vi "DAQStartRec.vi"(4 "entrée d'erreur (pas d'erreur)":errorcluster, 6 "ConfigurationTotale":T1, 7 "path out":path) -> (0 "sortie d'erreur":errorcluster, 3 "Refnum en sortie":refnum<k21>)   [LabVIEW 2015]
uses:
  DefDeType/ConfigTotale.ctl
  DefDeType/VoltageChannels.ctl
  DefDeType/WBridgeChannels.ctl
  DefDeType/Configuration.ctl
  <vilib>/DAQmx/configure/task.llb/DAQmx Configure Logging (TDMS).vi
  <vilib>/DAQmx/configure/trigger.llb/DAQmx Start Trigger (Digital Edge).vi
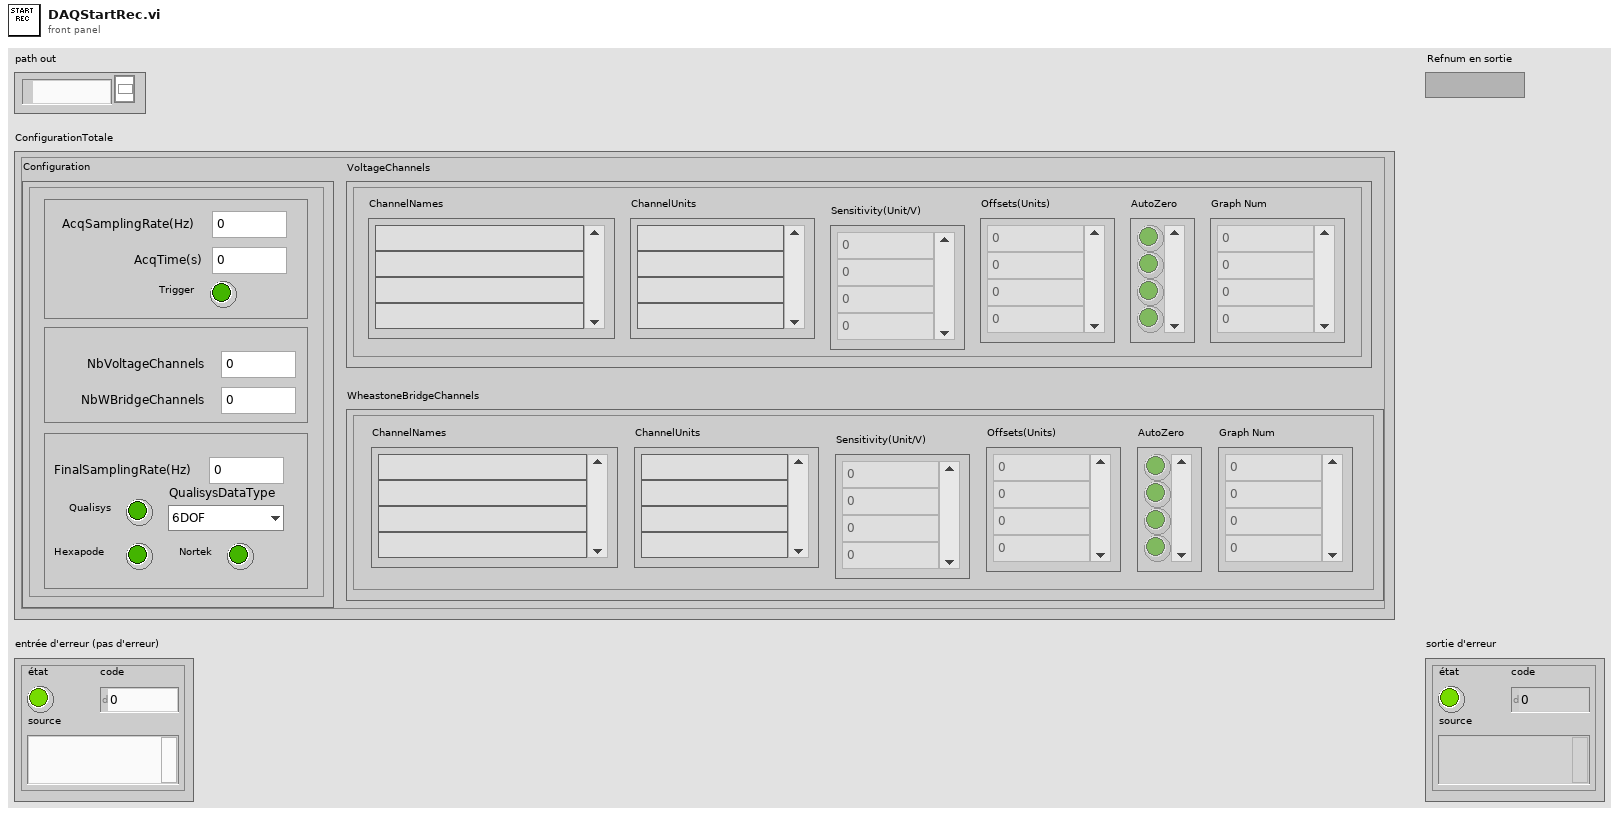
[diagram p1: front panel]
types:
  T1 = typedef "ConfigTotale.ctl" = cluster{"VoltageChannels":T2, "WheastoneBridgeChannels":T3, "Configuration":T4}
  T2 = typedef "VoltageChannels.ctl" = cluster{"ChannelNames":string[], "Sensitivity(Unit/V)":dbl[], "AutoZero":bool[], "ChannelUnits":string[], "Offsets(Units)":dbl[], "Graph Num":u8[]}
  T3 = typedef "WBridgeChannels.ctl" = cluster{"ChannelNames":string[], "Sensitivity(Unit/V)":dbl[], "AutoZero":bool[], "ChannelUnits":string[], "Offsets(Units)":dbl[], "Graph Num":u8[]}
  T4 = typedef "Configuration.ctl" = cluster{"AcqSamplingRate(Hz)":u32, "AcqTime(s)":u32, "Trigger":bool, "NbVoltageChannels":u32, "NbWBridgeChannels":u32, "Qualisys":bool, "Hexapode":bool, "FinalSamplingRate(Hz)":u32, "QualisysDataType":enum16{"6DOF", "3DTracking"}, "Nortek":bool}
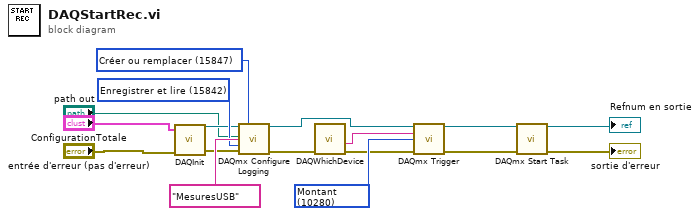
[diagram p0: block diagram]
diagram:
  w16 = 10280 items=["Montant"=10280, "Descendant"=10171] ("edge")
  w8 = 15847 items=["Ouvrir"=10437, "Ouvrir ou créer"=15846, "Créer ou remplacer"=15847, "Créer"=15848] ("operation")
  w7 = 15842 items=["Off"=10231, "Enregistrer"=15844, "Enregistrer et lire"=15842] ("logging mode")
  n1 = call "DAQInit.vi"("error in"="entrée d'erreur (pas d'erreur)", "configInput"="ConfigurationTotale") -> ("error out"=w5:errorcluster, "task out"=w6:refnum<k21>)  [unwired: 2 in]
  n2 = call-poly <vilib>:"DAQmx Configure Logging.vi"("task/channels in"=w6, "operation"=w8, "file path"="path out", "group name"="MesuresUSB", "logging mode"=w7, "error in"=w5) -> ("task out"=w10:refnum<k21>, "error out"=w9:errorcluster)  [unwired: 8 in]
  n3 = call "DAQWhichDevice.vi"("error in"=w9) -> ("error out"=w14:errorcluster, "sourceTrig"=w15:tag)  [unwired: 1 in, 5 out]
  n4 = call-poly <vilib>:"DAQmx Trigger.vi"("task/channels in"=w10, "source"=w15, "edge"=w16, "error in"=w14) -> ("task out"=w12:refnum<k21>, "error out"=w11:errorcluster)  [unwired: 10 in]
  n5 = call <vilib>:"DAQmx Start Task.vi"("task/channels in"=w12, "error in"=w11) -> ("task out"=→"Refnum en sortie":refnum<k21>, "error out"=→"sortie d'erreur":errorcluster)  [unwired: 12 in]
